vi "niFpgaTriggerTemplate.vi"(0 "trigger signal":fxp<+/-,16,16>, 1 "reset":bool, 7 "trigger type":enum8{"rising", "falling", "either"}(ring)) -> (4 "triggered":bool)   [LabVIEW 2017]
doc: "Detects changes of the input signal during a control or simulation process. The data type you wire to <B>trigger signal</B> determines the <B>triggered</B> data type."
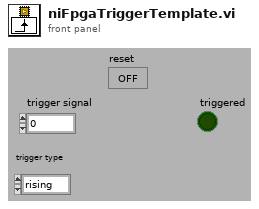
[diagram p1: front panel]
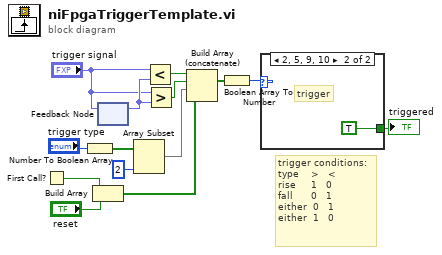
[diagram p0: block diagram]
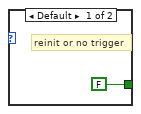
[diagram p2: hidden frame]
diagram:
  # "trigger conditions:\ntype    >   <\nrise     1   0\nfall      0   1\neither  0   1\neither  1   0"
  n1 = First Call?() -> (First Call?: T/F=w12:bool)
  n2 = Number To Boolean Array(number="trigger type") -> (Boolean array=w13:bool[])
  n3 = Build Array(w12, "reset") -> (w1:bool[])
  n4 = feedback-in #1("trigger signal") -> ()
  n5 = feedback #1() -> (w10:fxp<+/-,16,16>)  [unwired: 1 in]
  n6 = Array Subset(array=w13, length=2) -> (w8:bool[])  [unwired: 1 in]
  n7 = Less?(x="trigger signal", y=w10) -> (x < y?=w7:bool)
  n8 = Greater?(x="trigger signal", y=w10) -> (0:w6:bool)
  n9 = Build Array (concatenate)(w7, w6, w8, w1) -> (w5:bool[])
  n10 = Boolean Array To Number(Boolean array=w5) -> (number=w4:u8)
  n11 = case shown="2, 5, 9, 10" w4 {
    tunnel: [FALSE TRUE] -> w3
    frame Default {
      # "reinit or no trigger"
    }
    frame 2, 5, 9, 10 {
      # "trigger"
    }
  }
  "triggered" <- w3
